vi "RW DS402 Drive Slaves.vi"(7 "R/W Case":T11, 8 "error in (no error)":errorcluster, 10 "Async in":T10, 11 "DS402 EtherCAT Slave In":T1 {"I/O Output Data"."BD Refs"."Data Reference" format="%.0x"; "I/O Input Data"."BD Refs"."Data Reference" format="%.0x"; "I/O Output Vars"."VS ref" format="%.0x"; "I/O Input Vars"."VS ref" format="%.0x"; "VS ref" format="%.0x"}) -> (0 "error out":errorcluster, 2 "Async out":T10, 3 "DS402 EtherCAT Slave Out":T1 {"I/O Output Data"."BD Refs"."Data Reference" format="%.0x"; "I/O Input Data"."BD Refs"."Data Reference" format="%.0x"; "I/O Output Vars"."VS ref" format="%.0x"; "I/O Input Vars"."VS ref" format="%.0x"; "VS ref" format="%.0x"})   [LabVIEW 2016, in "Scan Engine Custom Device.lvlib"]
uses:
  Scan Engine Custom Device.lvlib
  Type Defs/RW Case.ctl
  Type Defs/Async Data.ctl
  Type Defs/Async Status.ctl
  Type Defs/Async State.ctl
  Type Defs/Async Command.ctl
  Type Defs/DS402 Drive ECAT Slave Data Cluster.ctl
  <vilib>/NI Veristand/Custom Device API/Custom Device Item Ref.ctl
  Type Defs/DS402 Drive ECAT Slave IOV Cluster.ctl
  Type Defs/UDV Data Type.ctl
  Type Defs/Input Data.ctl
  <vilib>/NI Veristand/Custom Device API/Block Data Reference.ctl
  <vilib>/NI Veristand/Custom Device API/Data Reference.ctl
  Type Defs/Output Data.ctl
  Type Defs/DS402 Drive ECAT Slave Action IOV Cluster.ctl
  Scanned Read - UDV.vi
  <vilib>/NI Veristand/Custom Device API/NI VeriStand - Set Channel Values by Block Data Reference.vi
  Scanned Write - UDV.vi
  <vilib>/NI Veristand/Custom Device API/NI VeriStand - Get Channel Values by Block Data Reference.vi
  <vilib>/NI Veristand/Custom Device API/Global Data Refs.vi
  <vilib>/NI Veristand/Custom Device API/Custom Device API.lvlib
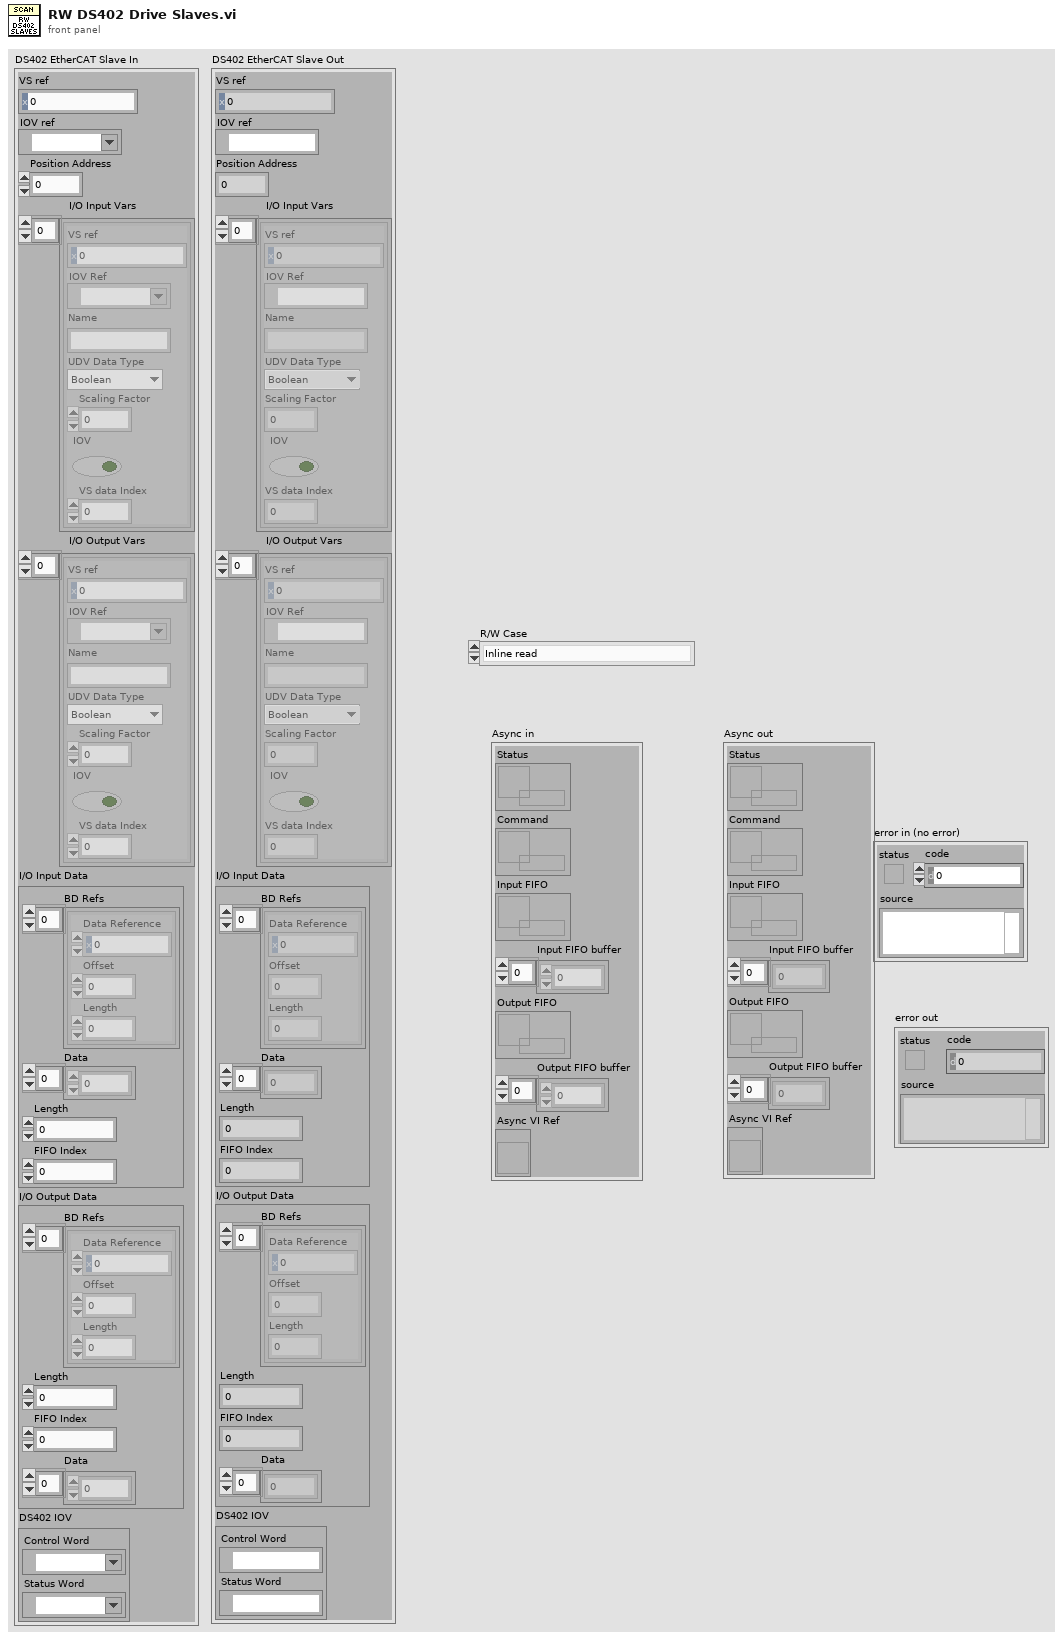
[diagram p1: front panel]
types:
  T1 = typedef "Scan Engine Custom Device.lvlib/DS402 Drive ECAT Slave Data Cluster.ctl" = cluster{"VS ref":T2, "IOV ref":refnum<k21>, "Position Address":u16, "I/O Input Vars ":T3[], "I/O Output Vars":T3[], "I/O Input Data":T5, "I/O Output Data":T8, "DS402 IOV":T9}
  T2 = typedef "Custom Device API.lvlib/Custom Device Item Ref.ctl" = u64
  T3 = typedef "Scan Engine Custom Device.lvlib/DS402 Drive ECAT Slave IOV Cluster.ctl" = cluster{"VS ref":T2, "IOV Ref":refnum<k21>, "Name":string, "UDV Data Type":T4, "Scaling Factor":dbl, "IOV":bool, "VS data Index":i32}
  T4 = typedef "Scan Engine Custom Device.lvlib/UDV Data Type.ctl" = enum16{"Boolean", "Fixed Point", "Int8", "Int16", "Int32", "Int64", "U32 Bit Field", "UInt8", "UInt16", "UInt32", "UInt64", "Other"}
  T5 = typedef "Scan Engine Custom Device.lvlib/Input Data.ctl" = cluster{"BD Refs":T6[], "Data":dbl[], "Length":i32, "FIFO Index":i32}
  T6 = typedef "Custom Device API.lvlib/Block Data Reference.ctl" = cluster{"Data Reference":T7, "Offset":u64, "Length":u64}
  T7 = typedef "Custom Device API.lvlib/Data Reference.ctl" = i32
  T8 = typedef "Scan Engine Custom Device.lvlib/Output Data.ctl" = cluster{"BD Refs":T6[], "Length":i32, "FIFO Index":i32, "Data":dbl[]}
  T9 = typedef "Scan Engine Custom Device.lvlib/DS402 Drive ECAT Slave Action IOV Cluster.ctl" = cluster{"Control Word":refnum<k21>, "Status Word":refnum<k21>}
  T10 = typedef "Scan Engine Custom Device.lvlib/Async Data.ctl" = cluster{"Status":refnum<queue>, "Command":refnum<queue>, "Input FIFO":refnum<k33>, "Input FIFO buffer":dbl[], "Output FIFO":refnum<k33>, "Output FIFO buffer":dbl[], "Async VI Ref":refnum<vi>}
  T11 = typedef "Scan Engine Custom Device.lvlib/RW Case.ctl" = enum16{"Inline read", "Inline write", "Async - Inline loop read", "Async - Inline loop write", "Async loop (read/write)"}
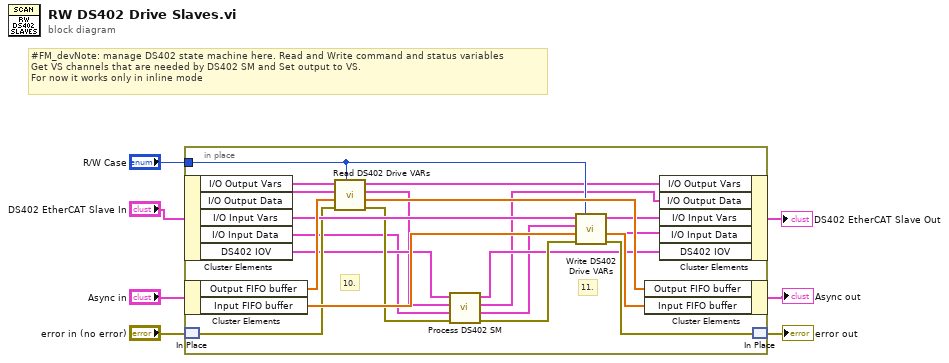
[diagram p0: block diagram]
diagram:
  # "#FM_devNote: manage DS402 state machine here. Read and Write command and status variables\nGet VS channels that are needed by DS402 SM and Set output to VS.\nFor now it works only in inline mode"
  n1 = in-place {
    in-place-border: "R/W Case" -> [w24]
    # "11."
    # "10."
    n2 = in-place-cluster #1("DS402 EtherCAT Slave In") -> ("I/O Output Vars"=w23:T3[], "I/O Output Data"=w19:T8, "I/O Input Vars"=w22:T3[], "I/O Input Data"=w9:T5, "DS402 IOV"=w13:T9)
    n3 = in-place-cluster #2("Async in") -> ("Output FIFO buffer"=w27:dbl[], "Input FIFO buffer"=w26:dbl[])
    n4 = in-place-match #3("error in (no error)") -> (w17:errorcluster)
    n5 = call "Read DS402 Drive VARs.vi"("R/W Case"=w24, "error in (no error)"=w17, "Output FIFO buffer in"=w27, "I/O Output Data In"=w19, "I/O Output Vars in"=w23) -> ("error out"=w15:errorcluster, "Output FIFO buffer out"=w28:dbl[], "I/O Output Data Out"=w11:T8, "I/O Output Vars out"=w21:T3[])  [unwired: 3 in]
    n6 = call "Process DS402 SM.vi"("error in (no error)"=w15, "I/O Input Data In"=w9, "I/O Output Data In"=w11, "DS402 IOV in"=w13) -> ("error out"=w14:errorcluster, "I/O Input Data Out"=w8:T5, "I/O Output Data Out"=w10:T8, "DS402 IOV out"=w12:T9)  [unwired: 4 in]
    n7 = call "Write DS402 Drive VARs.vi"("R/W Case"=w24, "error in (no error)"=w14, "Input FIFO buffer in"=w26, "I/O Input Data In"=w8, "I/O Imput Vars in"=w22) -> ("error out"=w16:errorcluster, "Input FIFO buffer out"=w25:dbl[], "I/O Input Data Out"=w18:T5, "I/O Imput Vars out"=w20:T3[])  [unwired: 3 in]
    n8 = in-place-cluster #2("Output FIFO buffer"=w28, "Input FIFO buffer"=w25) -> (→"Async out":T10)
    n9 = in-place-cluster #1("I/O Output Vars"=w21, "I/O Output Data"=w10, "I/O Input Vars"=w20, "I/O Input Data"=w18, "DS402 IOV"=w12) -> (→"DS402 EtherCAT Slave Out":T1)
    n10 = in-place-match #3(w16) -> (→"error out":errorcluster)
  }
